vi "Open Connection.vi"(8 "error in (no error)":errorcluster, 10 "Connection":refnum<class "Database Connection.lvclass">, 11 "ADODB in":refnum<class "ADODB.lvclass">) -> (0 "error out":errorcluster, 3 "ADODB out":refnum<class "ADODB.lvclass">)   [LabVIEW 2020, in "ADODB.lvlib" / "ADODB.lvclass"]
uses:
  ADODB.lvclass
  Database Interfaces/Database Connection Class/Database Connection.lvclass
  UDL Connection Class/UDL Connection.lvclass
  MS Access Database Engine/MS Access Database Engine.lvclass
  C:/Users/User/Desktop/Raman Program/Database OOP/source/Database OOP/Database Libraries/DBMS Specific/DBMS Specific.lvclass
  ADODB.lvclass/ADODB.ctl
  <vilib>/addons/database/Connection.llb/DB Tools Open Connec (Path).vi
  <vilib>/addons/database/NI_Database_API.lvlib
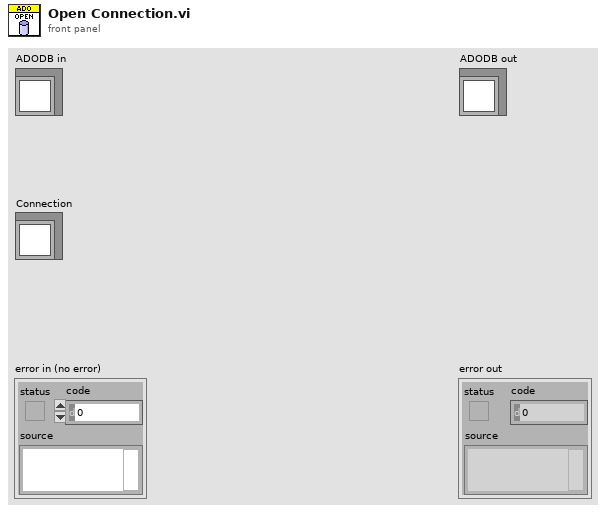
[diagram p1: front panel]
types:
  T1 = typedef "NI_Database_API.lvlib/Conn ObjectReference.ctl" = refnum<k1>
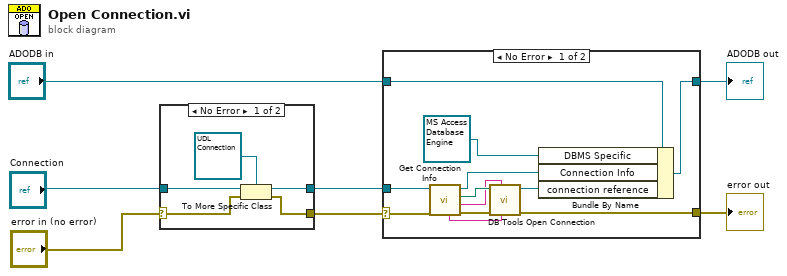
[diagram p0: block diagram]
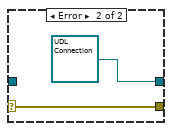
[diagram p2: hidden frame]
diagram:
  n1 = case shown="No Error" "error in (no error)" {
    selector: "error in (no error)" -> [w9 w14]
    tunnel: "Connection" -> [w12 _]
    tunnel: [w11 w14] -> w3
    tunnel: [w8 refnum<class "UDL Connection.lvclass"> refnum ("ADODB.lvlib:UDL Connection.lvclass")] -> w1
    frame No Error {
      n2 = To More Specific Class(target class=refnum<class "UDL Connection.lvclass"> refnum ("ADODB.lvlib:UDL Connection.lvclass"), reference=w12, error in=w9) -> (specific class reference=w8:refnum<class "UDL Connection.lvclass">, error out=w11:errorcluster)
    }
    frame Error {
    }
  }
  n3 = case shown="No Error" w3 {
    selector: w3 -> [w21 w28]
    tunnel: [w24 w28] -> w7
    tunnel: "ADODB in" -> [w26 w27]
    tunnel: [w25 w27] -> w5
    tunnel: w1 -> [w22 _]
    frame No Error {
      n4 = call-dynamic "Get Connection Info.vi"("error in (no error)"=w21, "UDL Connection in"=w22) -> ("error out"=w20:errorcluster, "User"=w17:string, "*.uld file path"=w18:path, "UDL Connection out"=w19:refnum<class "UDL Connection.lvclass">, "Password"=w16:string)  [unwired: 5 in]
      n5 = call-poly <vilib>:"DB Tools Open Connection.vi"("password"=w16, "userID"=w17, "error in (no error)"=w20, "connection information"=w18) -> ("error out"=w24:errorcluster, "connection reference"=w23:T1)  [unwired: 4 in]
      n6 = Bundle By Name(cluster=w26, "DBMS Specific"=refnum<class "MS Access Database Engine.lvclass"> refnum ("ADODB.lvlib:MS Access Database Engine.lvclass"), "Connection Info"=w19, "connection reference"=w23) -> (w25:refnum<class "ADODB.lvclass">)
    }
    frame Error {
    }
  }
  "error out" <- w7
  "ADODB out" <- w5
